vi "CloseMenu.vi"(8 "error in (no error)":errorcluster, 11 "Game in":refnum<class "Game.lvclass">) -> (0 "error out":errorcluster, 3 "Game out":refnum<class "Game.lvclass">)   [LabVIEW 2019, in "RT_Game.lvlib" / "Game.lvclass"]
uses:
  Game.lvclass
  Game.lvclass/Game.ctl
  Menu/States.ctl
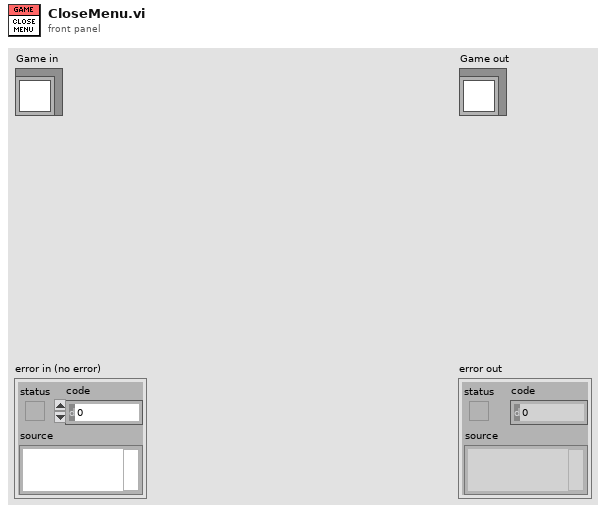
[diagram p1: front panel]
types:
  T1 = typedef "RT_Game.lvlib/Game.lvclass/States.ctl" = enum16{"Init", "Restart", "Menu", "Game", "Resume", "ToggleSingleplayer", "LoadNextGame", "ExitToMenu", "NewHighscore", "GameOver", "SlideOut"}
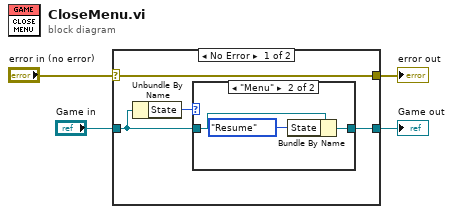
[diagram p0: block diagram]
diagram:
  n1 = case shown="No Error" "error in (no error)" {
    selector: "error in (no error)" -> [w8 w14]
    tunnel: [w8 w14] -> w3
    tunnel: [w7 w13] -> w1
    tunnel: "Game in" -> [w6 w13]
    frame No Error {
      n2 = Unbundle By Name(w6) -> ("State"=w5:T1)
      n3 = case shown="\"Menu\"" w5 {
        tunnel: w6 -> [w9 w12]
        tunnel: [w9 w11] -> w7
        frame "Init", Default {
        }
        frame "Menu" {
          n4 = Bundle By Name(cluster=w12, "State"=States."Resume") -> (w11:refnum<class "Game.lvclass">)
        }
      }
    }
    frame Error {
    }
  }
  "error out" <- w3
  "Game out" <- w1
